vi "Cornerstone_Query.vi"(8 "error in":errorcluster, 10 "Query":string, 11 "VISA resource IN":refnum<visa-resource-name>) -> (0 "error out":errorcluster, 2 "Read Data":string, 3 "VISA resource OUT":refnum<visa-resource-name>)   [LabVIEW 2017]
doc: "This VI is for sending a command and receiving response from the Cornerstone Monochromator."
panel:
  # "Written by Kyle Montgomery, PhD\nVisit: kmontgomery.net"
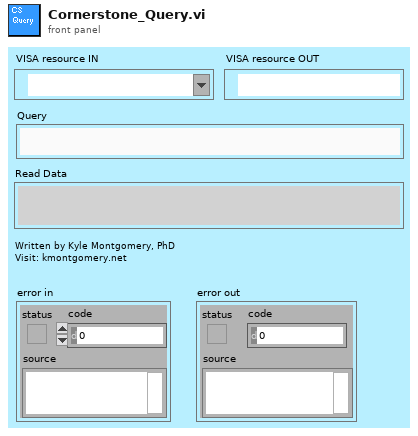
[diagram p1: front panel]
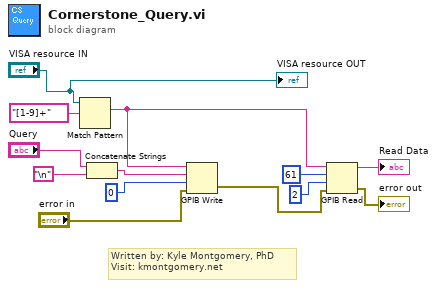
[diagram p0: block diagram]
diagram:
  # "Written by: Kyle Montgomery, PhD\nVisit: kmontgomery.net"
  n1 = Match Pattern(string="VISA resource IN", regular expression="[1-9]+") -> (match substring=w3:string)  [unwired: 4 out]
  n2 = Concatenate Strings("Query", "\n") -> (w10:string)
  n3 = GPIB Write(0:w3, 1:w10, 2:i16 0 ("mode (0)"), 3:"error in") -> (6:w4:errorcluster)  [unwired: 2 out]
  n4 = GPIB Read(0:w3, 1:61 ("byte count"), 2:i16 2 ("mode (0)"), 3:w4) -> (5:→"Read Data":string, 7:→"error out":errorcluster)  [unwired: 2 out]
  "VISA resource OUT" <- "VISA resource IN"
